vi "YH_guanli.vi"(0 "action":string, 1 "LabVIEW Web Service Request":refnum<class "Web Request.lvclass"> caption="LabVIEW Web服务请求", 2 "key":string, 3 "juese":string, 4 "beizhu":string, 5 "id":string, 7 "gonghao":string, 8 "didian":string, 9 "name":string, 11 "number":string, 13 "sjbumen":string, 14 "psw":string) -> (10 "error":errorcluster)   [LabVIEW 2017]
uses:
  <vilib>/wsapi/Web Request.lvclass
panel:
  out "postdata":string caption="post数据"
  out "error out":errorcluster caption="错误输出"
  # "Web服务请求输入接线端用于调用“Web服务”选板的VI。除非不需要访问该选板，否则不要在连线板上删除这个输入接线端。"
  # "添加至连线板的每一个其他输入控件，在URL中对应于一个输入。如需在接线端模式输出（默认设置）下包含显示控件，则该显示控件必须与连线板相连。"
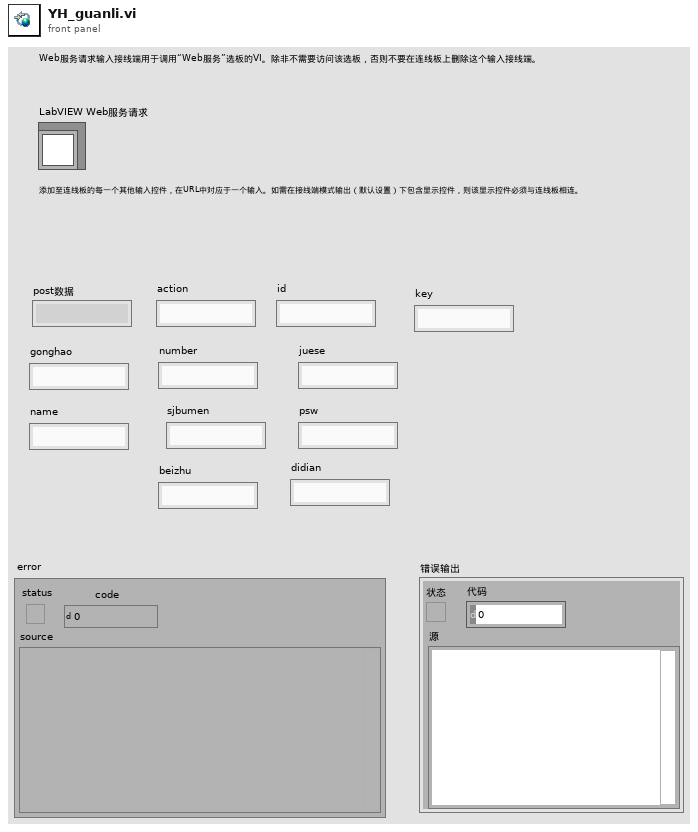
[diagram p1: front panel]
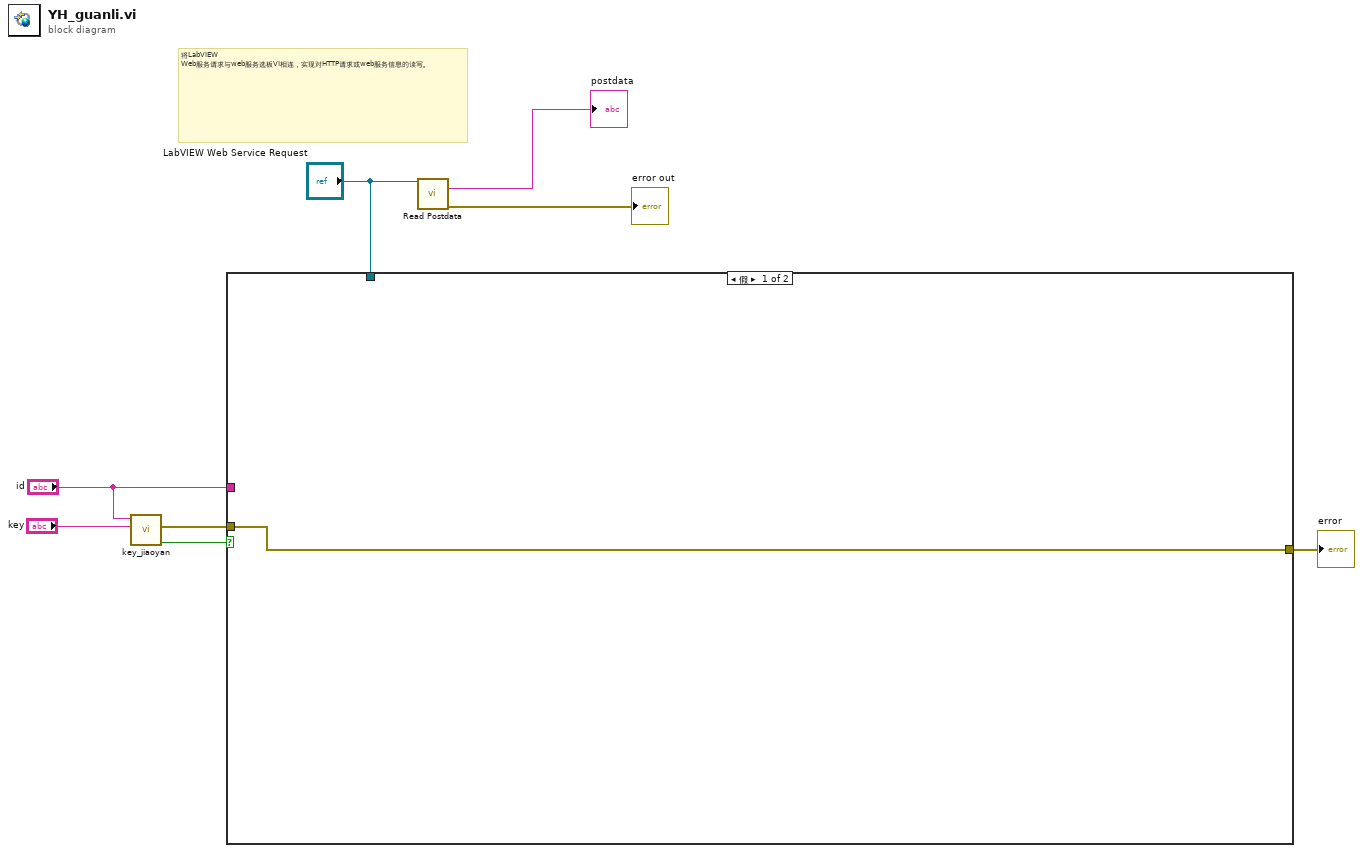
[diagram p0: block diagram]
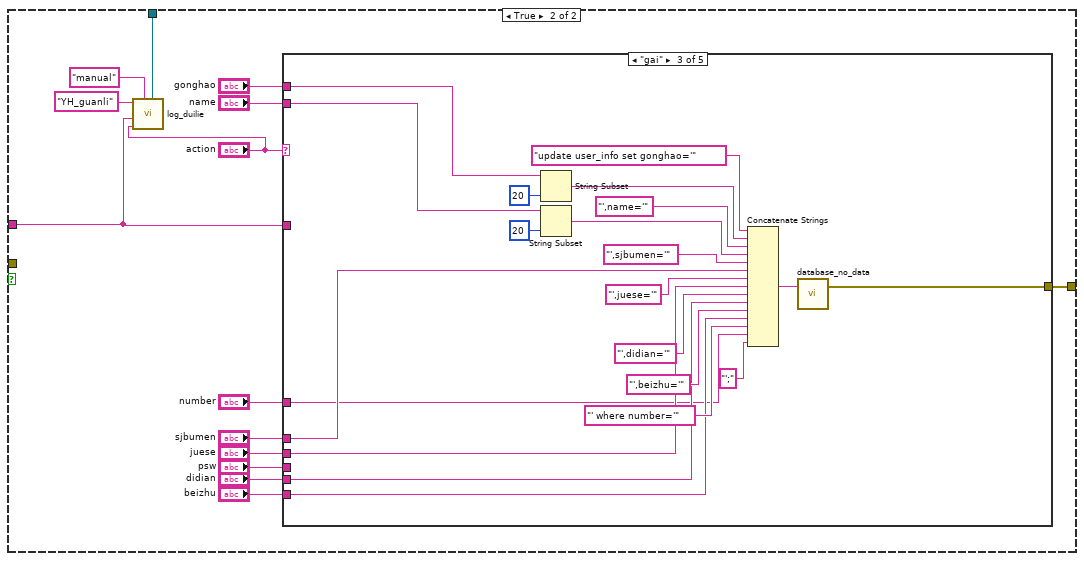
[diagram p2: hidden frame]
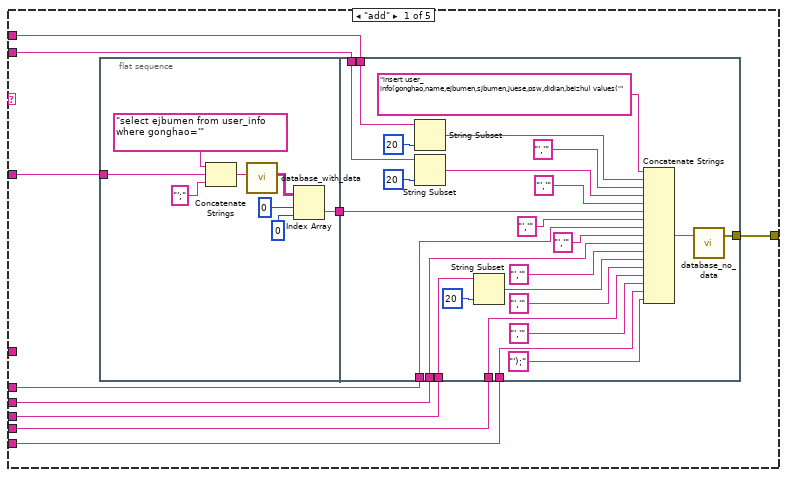
[diagram p3: hidden frame]
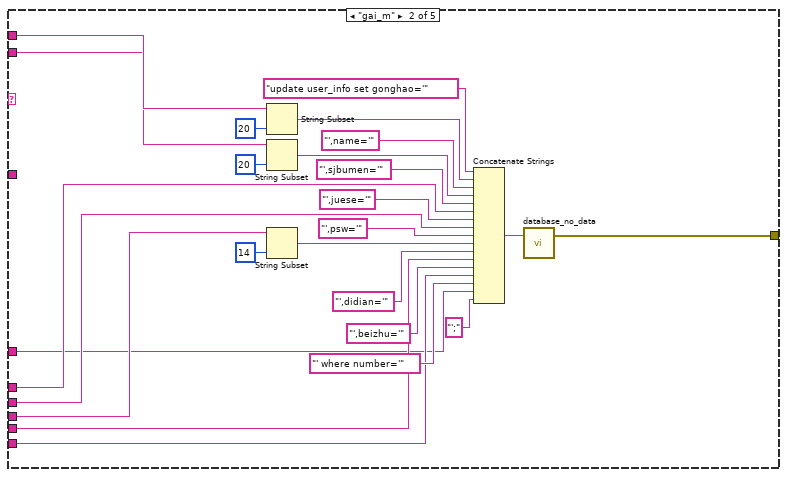
[diagram p4: hidden frame]
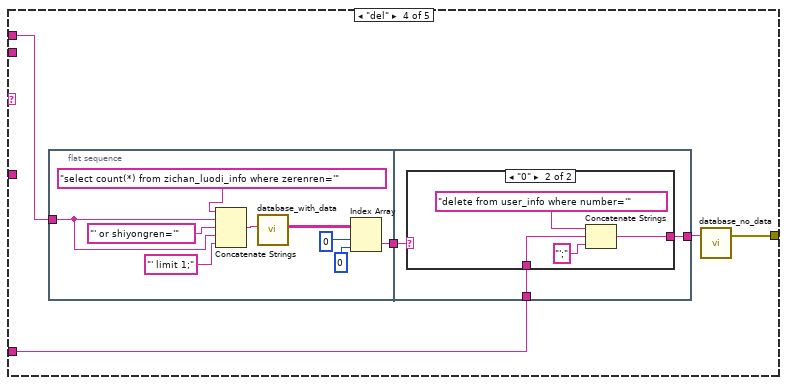
[diagram p5: hidden frame]
diagram:
  # "将LabVIEW Web服务请求与web服务选板VI相连，实现对HTTP请求或web服务信息的读写。"
  n1 = call "key_jiaoyan.vi"("key_client"="key", "gonghao"="id") -> ("jy"=w2:bool, "error"=w1:errorcluster)  [unwired: 8 in]
  n2 = case shown="假" w2 {
    tunnel: [w9 w23] -> w7
    tunnel: "LabVIEW Web Service Request" -> [_ w14]
    tunnel: "id" -> [_ w10]
    tunnel: w1 -> [w9 _]
    frame False {
    }
    frame True {
      n3 = call "log_duilie.vi"("LabVIEW Web Service Request"=w14, "type"="manual", "action"="action", "user"=w10, "yw"="YH_guanli") -> ()  [unwired: 7 in]
      n4 = case shown="\"gai\"" "action" {
        tunnel: [w33 w75 w99 w117 _] -> w23
        tunnel: "didian" -> [w31 w69 w94 _ _]
        tunnel: "psw" -> [w30 w70 _ _ _]
        tunnel: "juese" -> [w29 w71 w95 _ _]
        tunnel: "sjbumen" -> [w26 w72 w96 _ _]
        tunnel: "name" -> [w28 w73 w97 _ _]
        tunnel: "gonghao" -> [w27 w74 w98 w114 _]
        tunnel: "beizhu" -> [w32 w68 w93 _ _]
        tunnel: w10 -> [w25 _ _ _ _]
        tunnel: "number" -> [_ w67 w92 w113 _]
        frame "add" {
          n5 = flat-sequence {
            tunnel: w25 -> [w40]
            tunnel: [w35] -> w24
            tunnel: [w51] -> w33
            tunnel: w32 -> [w50]
            tunnel: w31 -> [w49]
            tunnel: w30 -> [w48]
            tunnel: w29 -> [w47]
            tunnel: w28 -> [w46]
            tunnel: w27 -> [w45]
            tunnel: w26 -> [w44]
            tunnel: w24 -> [w42]
            frame #0 {
              n6 = Concatenate Strings("select ejbumen from user_info where gonghao='" ("字符串"), w40, "';" ("字符串")) -> (w39:string)
              n7 = call "database_with_data.vi"("input"=w39) -> ("Data"=w36:string[][])  [unwired: 9 in, 1 out]
              n8 = Index Array(array=w36, index (row)=0 ("索引 (行)"), index (col)=0 ("禁用的索引 (列)")) -> (element=w35:string)
            }
            frame #1 {
              n9 = String Subset(string=w45, length (rest)=20 ("长度（剩余）")) -> (substring=w64:string)  [unwired: 1 in]
              n10 = String Subset(string=w46, length (rest)=20 ("长度（剩余）")) -> (substring=w62:string)  [unwired: 1 in]
              n11 = String Subset(string=w48, length (rest)=20 ("长度（剩余）")) -> (substring=w53:string)  [unwired: 1 in]
              n12 = Concatenate Strings("insert user_info(gonghao,name,ejbumen,sjbumen,juese,psw,didian,beizhu) values('" ("格式字符串"), w64, "','" ("字符串"), w62, "','" ("字符串"), w42, "','" ("字符串"), w44, "','" ("字符串"), w47, "','" ("字符串"), w53, "','" ("字符串"), w49, "','" ("字符串"), w50, "');" ("字符串")) -> (w52:string)
              n13 = call "database_no_data.vi"("input"=w52) -> ("error"=w51:errorcluster)  [unwired: 2 in]
            }
          }
        }
        frame "gai_m" {
          n14 = String Subset(string=w74, length (rest)=20 ("长度（剩余）")) -> (substring=w88:string)  [unwired: 1 in]
          n15 = String Subset(string=w73, length (rest)=20 ("长度（剩余）")) -> (substring=w89:string)  [unwired: 1 in]
          n16 = String Subset(string=w70, length (rest)=14 ("长度（剩余）")) -> (substring=w91:string)  [unwired: 1 in]
          n17 = Concatenate Strings("update user_info set gonghao='" ("格式字符串"), w88, "',name='" ("字符串"), w89, "',sjbumen='" ("字符串"), w72, "',juese='" ("字符串"), w71, "',psw='" ("字符串"), w91, "',didian='" ("字符串"), w69, "',beizhu='" ("字符串"), w68, "' where number='" ("字符串"), w67, "';" ("字符串")) -> (w90:string)
          n18 = call "database_no_data.vi"("input"=w90) -> ("error"=w75:errorcluster)  [unwired: 2 in]
        }
        frame "gai" {
          n19 = String Subset(string=w98, length (rest)=20 ("长度（剩余）")) -> (substring=w110:string)  [unwired: 1 in]
          n20 = String Subset(string=w97, length (rest)=20 ("长度（剩余）")) -> (substring=w111:string)  [unwired: 1 in]
          n21 = Concatenate Strings("update user_info set gonghao='" ("格式字符串"), w110, "',name='" ("字符串"), w111, "',sjbumen='" ("字符串"), w96, "',juese='" ("字符串"), w95, "',didian='" ("字符串"), w94, "',beizhu='" ("字符串"), w93, "' where number='" ("字符串"), w92, "';" ("字符串")) -> (w112:string)
          n22 = call "database_no_data.vi"("input"=w112) -> ("error"=w99:errorcluster)  [unwired: 2 in]
        }
        frame "del" {
          n23 = flat-sequence {
            tunnel: w114 -> [w119]
            tunnel: [w121] -> w116
            tunnel: [w129] -> w115
            tunnel: w116 -> [w128]
            tunnel: w113 -> [w127]
            frame #0 {
              n24 = Concatenate Strings("select count(*) from zichan_luodi_info where zerenren='" ("格式字符串"), w119, "' or shiyongren='" ("字符串"), w119, "' limit 1;" ("字符串")) -> (w125:string)
              n25 = call "database_with_data.vi"("input"=w125) -> ("Data"=w122:string[][])  [unwired: 9 in, 1 out]
              n26 = Index Array(array=w122, index (row)=0 ("索引 (行)"), index (col)=0 ("禁用的索引 (列)")) -> (element=w121:string)
            }
            frame #1 {
              n27 = case shown="\"0\"" w128 {
                tunnel: [_ w131] -> w129
                tunnel: w127 -> [_ w130]
                frame "假", Default {
                }
                frame "0" {
                  n28 = Concatenate Strings("delete from user_info where number='" ("格式字符串"), w130, "';" ("字符串")) -> (w131:string)
                }
              }
            }
          }
          n29 = call "database_no_data.vi"("input"=w115) -> ("error"=w117:errorcluster)  [unwired: 2 in]
        }
        frame Default {
        }
      }
    }
  }
  "error" <- w7
  n30 = call <vilib>:"Read Postdata.vi"("LabVIEW Web Service Request"="LabVIEW Web Service Request") -> ("postdata"=→"postdata":string, "error out"=→"error out":errorcluster)  [unwired: 12 in, 1 out]
